vi "PLL_Simple_WithoutTime.vi"() -> ()   [LabVIEW 2019]
uses:
  <vilib>/Analysis/NI_AALBase.lvlib
panel:
  out "Waveform Graph":dbl[][](graph)
  in  "Reset":bool
  in  "stop":bool
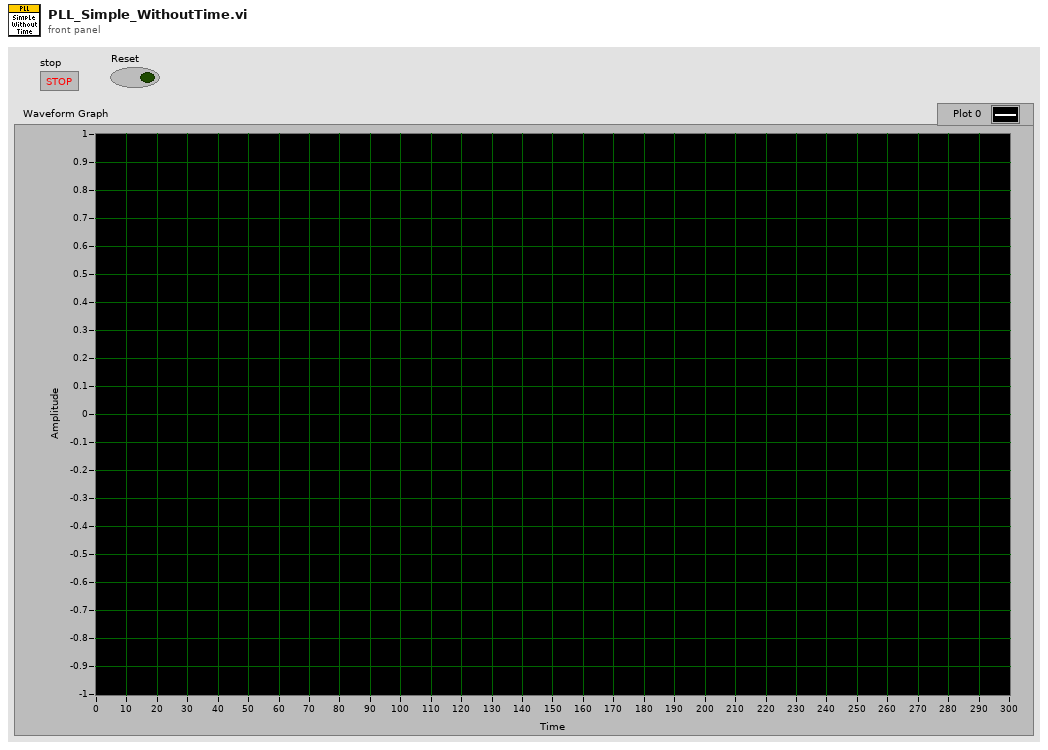
[diagram p1: front panel]
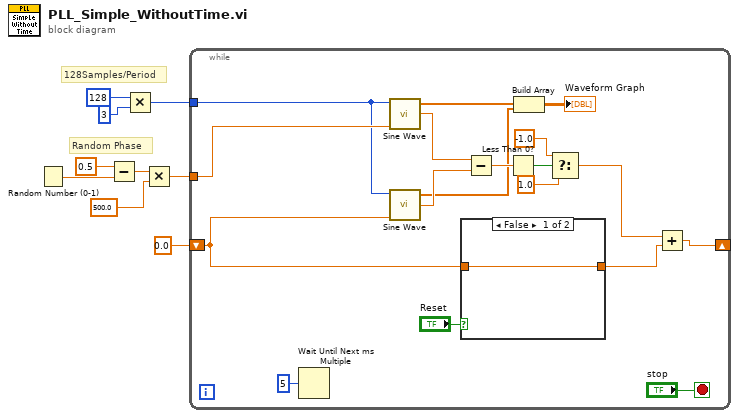
[diagram p0: block diagram]
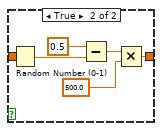
[diagram p2: hidden frame]
diagram:
  # "128Samples/Period"
  # "Random Phase"
  n1 = Random Number (0-1)() -> (number: 0 to 1=w9:dbl)
  n2 = Subtract(x=0.5, y=w9) -> (x-y=w7:dbl)
  n3 = Multiply(x=128, y=3) -> (x*y=w3:i32)
  n4 = Multiply(x=w7, y=500.0) -> (x*y=w5:dbl)
  n5 = while {
    tunnel: w3 -> [w24]
    tunnel: w5 -> [w25]
    shift-right: [w16] -> _
    shift-left: 0.0 -> [w11]
    stop <- "stop" stop-if-true
    n6 = Wait Until Next ms Multiple(millisecond multiple=u32 5) -> ()  [unwired: 1 out]
    n7 = call <vilib>:"Sine Wave.vi"("samples"=w24, "phase in"=w25) -> ("sine wave"=w15:dbl[], "phase out"=w23:dbl)  [unwired: 3 in, 1 out]
    n8 = call <vilib>:"Sine Wave.vi"("samples"=w24, "phase in"=w11) -> ("sine wave"=w14:dbl[], "phase out"=w22:dbl)  [unwired: 3 in, 1 out]
    n9 = case shown="False" "Reset" {
      tunnel: [w28 w29] -> w12
      tunnel: w11 -> [w28 _]
      frame False {
      }
      frame True {
        n10 = Random Number (0-1)() -> (number: 0 to 1=w30:dbl)
        n11 = Subtract(x=0.5, y=w30) -> (x-y=w32:dbl)
        n12 = Multiply(x=w32, y=500.0) -> (x*y=w29:dbl)
      }
    }
    n13 = Subtract(x=w23, y=w22) -> (x-y=w21:dbl)
    n14 = Less Than 0?(x=w21) -> (x < 0?=w20:bool)
    n15 = Build Array(w15, w14) -> (→"Waveform Graph":dbl[][])
    n16 = Select(t=-1.0, s=w20, f=1.0) -> (s? t:f=w17:dbl)
    n17 = Add(x=w17, y=w12) -> (x+y=w16:dbl)
  }
